vi "Read Start Homing.vi"(8 "error in (no error)":errorcluster, 11 "FHPP in":refnum<class "FHPP.lvclass">) -> (0 "error out":errorcluster, 2 "Start":bool, 3 "FHPP out":refnum<class "FHPP.lvclass">)   [LabVIEW 2022 SP3, in "FHPP.lvclass"]
uses:
  FHPP.lvclass
  FHPP.lvclass/FHPP.ctl
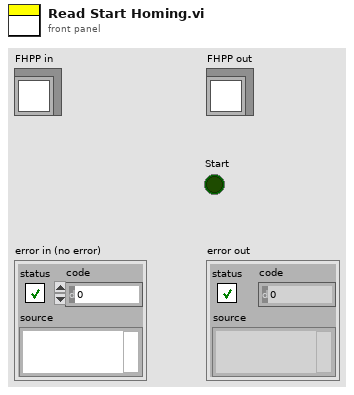
[diagram p1: front panel]
types:
  T1 = typedef "FHPP.lvclass/CPOS.ctl" = cluster{"Halt":bool, "Start":bool, "Start Homing":bool, "Jog Positive":bool, "Jog Negative":bool, "Teach Actual Value":bool, "Clear Remaining Pos":bool, "Reserved":bool}
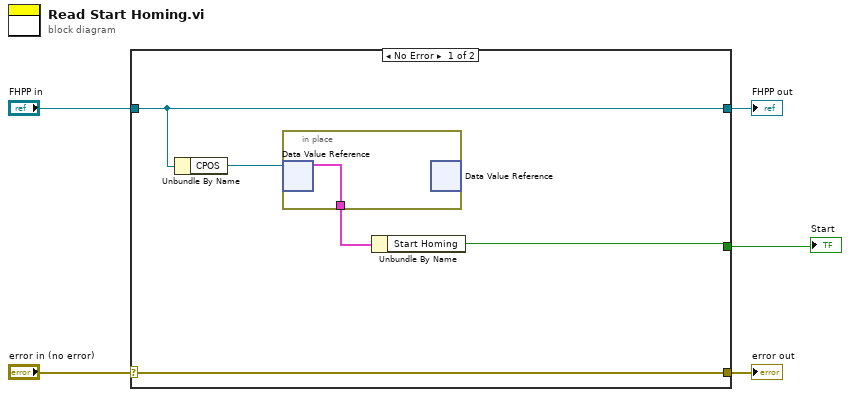
[diagram p0: block diagram]
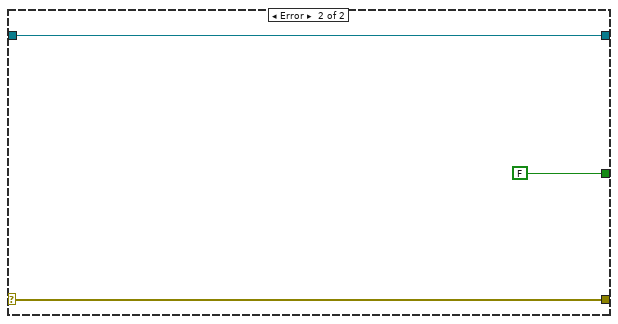
[diagram p2: hidden frame]
diagram:
  n1 = case shown="No Error" "error in (no error)" {
    selector: "error in (no error)" -> [w10 w14]
    tunnel: [w10 w14] -> w4
    tunnel: [w9 w13] -> w2
    tunnel: "FHPP in" -> [w9 w13]
    tunnel: [w6 FALSE] -> w1
    frame No Error {
      n2 = Unbundle By Name(w9) -> ("CPOS"=w8:refnum<data-value>)
      n3 = in-place {
        in-place-border: [w11] -> w7
        n4 = in-place-dvr #1(w8) -> (w11:T1)  [unwired: 1 out]
        n5 = in-place-dvr #1() -> ()  [unwired: 1 in, 2 out]
      }
      n6 = Unbundle By Name(w7) -> ("Start Homing"=w6:bool)
    }
    frame Error {
    }
  }
  "error out" <- w4
  "FHPP out" <- w2
  "Start" <- w1
